vi "Shooter_SM.vi"   [LabVIEW 2017]
uses:
  Enum_Shooter_SM_State.ctl
  Enum_Shooter_SM_Action.ctl
  Globals/Global_STOP.vi
  Global_HoodSensorPosition.vi
  Global_CMDShooter.vi
  Global_ShooterCTRL.vi
  Enum_ShooterCMDS.ctl
  Cluster_ShooterCMDInput.ctl
  Vision/Enum_ Field Targets.ctl
  Vision/ENUM_Location Zones.ctl
  Vision/Cluster_HW Data Out.ctl
  Vision/Global_HW Data Out.vi
types:
  T1 = typedef "Vision.lvlib/Cluster_HW Data Out.ctl" = cluster{"Target Found":bool, "Target":T2, "Nominal to Center (-1to1":dbl, "Pixels to Center":dbl, "Vision Distance (in)":dbl, "Location":T3}
  T2 = typedef "Vision.lvlib/Enum_ Field Targets.ctl" = enum16{"None", "Peg", "Boiler", "Rope"}
  T3 = typedef "Vision.lvlib/ENUM_Location Zones.ctl" = enum16{"Unknown", "Close", "Medium-Close", "Medium", "Medium -Far", "Far"}
  T4 = typedef "Cluster_ShooterCMDInput.ctl" = cluster{"Fly Wheel Input":dbl, "Hood position Input":dbl, "CMD Mode":T5}
  T5 = typedef "Enum_ShooterCMDS.ctl" = enum16{"Shooting", "Not Shooting"}
  T6 = typedef "Enum_Shooter_SM_Action.ctl" = enum16{"No Action", "Reset Time", "Reset All", "Set Hood", "Set Fly Wheel", "Stop Hood"}
  T7 = typedef "Enum_Shooter_SM_State.ctl" = enum16{"Startup", "Idle", "Shutdown", "Check Position"}
  T8 = cluster{"Action":T6[], "State":T7, "Current Time":timestamp, "Start Time":timestamp, "Loop Time (ms)":u32, "Hood Position Out":dbl, "Fly Wheel Out":dbl, "Hood Sensor Position":dbl, "Shooter CMD":T4, "Hood VBus Out":dbl, "Hood Pos/Vbus":bool, "Tracking Data OUT":T1}
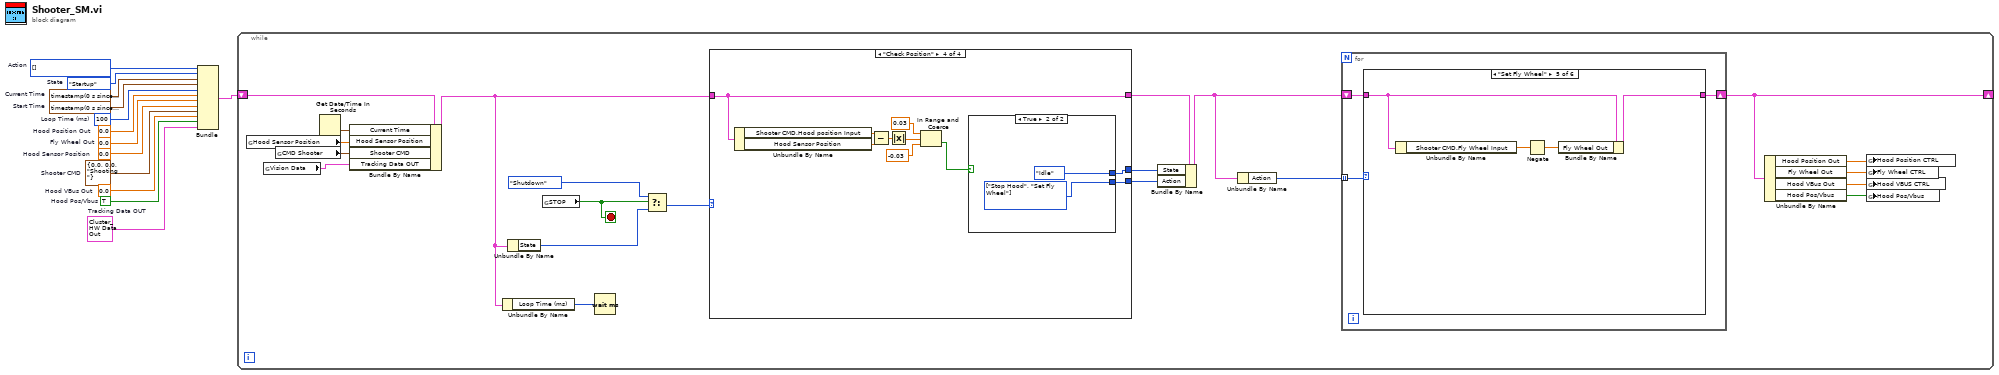
[diagram p0: block diagram]
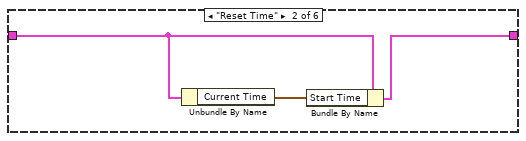
[diagram p3: hidden frame]
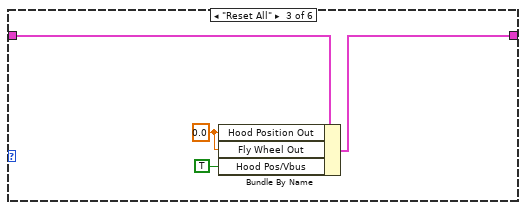
[diagram p4: hidden frame]
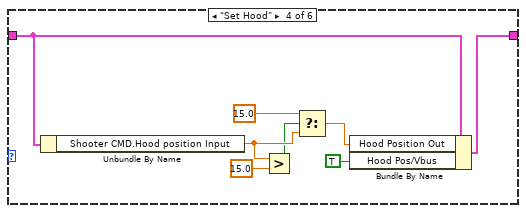
[diagram p5: hidden frame]
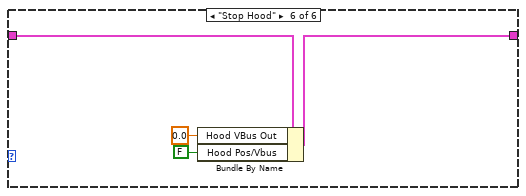
[diagram p6: hidden frame]
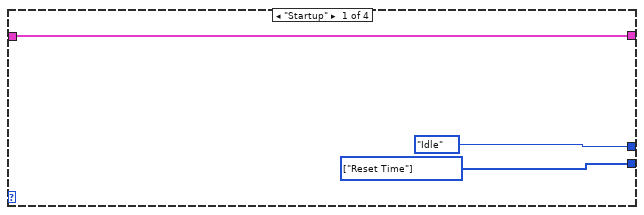
[diagram p7: hidden frame]
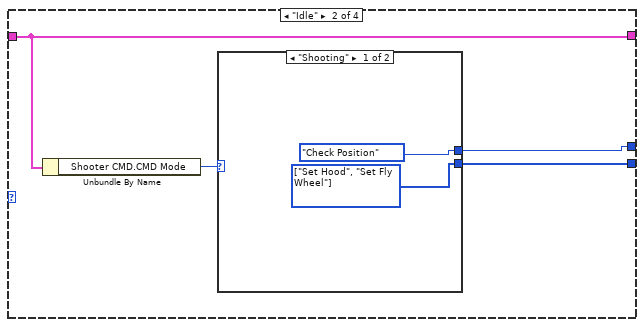
[diagram p8: hidden frame]
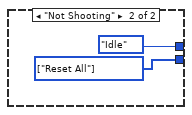
[diagram p9: hidden frame]
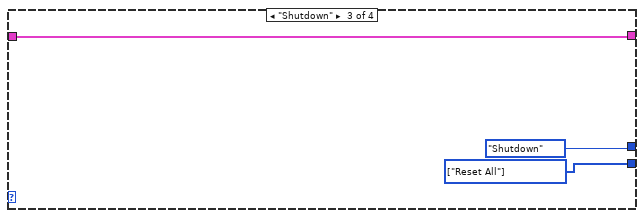
[diagram p10: hidden frame]
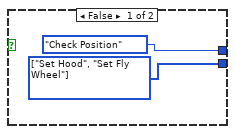
[diagram p11: hidden frame]
diagram:
  w1 = T1 {"Target Found"=FALSE, "Target"=enum."None", "Nominal to Center (-1to1"=0.0, "Pixels to Center"=0.0, "Vision Distance (in)"=0.0, "Location"=enum."Unknown"}  # Tracking Data OUT
  w13 = TRUE  # Hood Pos/Vbus
  w12 = 0.0  # Hood VBus Out
  w11 = T4 {"Fly Wheel Input"=0.0, "Hood position Input"=0.0, "CMD Mode"=enum."Shooting"}  # Shooter CMD
  w10 = 0.0  # Hood Sensor Position
  w9 = 0.0  # Fly Wheel Out
  w8 = 0.0  # Hood Position Out
  w7 = T6[] [] items=["No Action", "Reset Time", "Reset All", "Set Hood", "Set Fly Wheel", "Stop Hood"]  # Action
  w6 = Enum_Shooter_SM_State."Startup"  # State
  w2 = u32 100  # Loop Time (ms)
  w3 = timestamp(0 s since 1904-01-01)  # Start Time
  w4 = timestamp(0 s since 1904-01-01)  # Current Time
  n1 = Bundle("Action"=w7, "State"=w6, "Current Time"=w4, "Start Time"=w3, "Loop Time (ms)"=w2, "Hood Position Out"=w8, "Fly Wheel Out"=w9, "Hood Sensor Position"=w10, "Shooter CMD"=w11, "Hood VBus Out"=w12, "Hood Pos/Vbus"=w13, "Tracking Data OUT"=w1) -> (w5:T8)  [unwired: 1 in]
  n2 = while {
    shift-right: [w21] -> _
    shift-left: w5 -> [w26]
    stop <- w33 stop-if-true
    n3 = global read "Global_HoodSensorPosition.vi" "Hood Sensor Position"() -> (w24:dbl)
    n4 = global read "Global_HW Data Out.vi" "Vision Data"() -> (w14:T1)
    n5 = global read "Global_CMDShooter.vi" "CMD Shooter"() -> (w22:T4)
    n6 = Get Date/Time In Seconds() -> (seconds since 1Jan1904=w23:timestamp)
    n7 = Bundle By Name(cluster=w26, "Current Time"=w23, "Hood Sensor Position"=w24, "Shooter CMD"=w22, "Tracking Data OUT"=w14) -> (w25:T8)
    n8 = Unbundle By Name(w25) -> ("Loop Time (ms)"=w30:u32)
    n9 = Unbundle By Name(w25) -> ("State"=w31:T7)
    n10 = global read "Global_Stop.vi" "STOP"() -> (w33:bool)
    n11 = Wait (ms)(milliseconds to wait=w30) -> ()  [unwired: 1 out]
    n12 = Select(t=Enum_Shooter_SM_State."Shutdown" ("Enum"), s=w33, f=w31) -> (s? t:f=w34:T7)
    n13 = case shown="\"Check Position\"" w34 {
      tunnel: w25 -> [w62 w66 w73 w85]
      tunnel: [w62 w66 w73 w85] -> w29
      tunnel: [Enum_Shooter_SM_State."Idle" ("State") w68 Enum_Shooter_SM_State."Shutdown" ("State") w77] -> w18
      tunnel: [w63 w67 w74 w76] -> w17
      frame "Startup" {
        w63 = T6[] [enum."Reset Time"] items=["No Action", "Reset Time", "Reset All", "Set Hood", "Set Fly Wheel", "Stop Hood"] ("Action")
      }
      frame "Idle" {
        n14 = Unbundle By Name(w66) -> ("Shooter CMD.CMD Mode"=w65:T5)
        n15 = case shown="\"Shooting\"" w65 {
          tunnel: [Enum_Shooter_SM_State."Check Position" ("State") Enum_Shooter_SM_State."Idle" ("State")] -> w68
          tunnel: [w69 w71] -> w67
          frame "Shooting" {
            w69 = T6[] [enum."Set Hood", enum."Set Fly Wheel"] items=["No Action", "Reset Time", "Reset All", "Set Hood", "Set Fly Wheel", "Stop Hood"] ("Action")
          }
          frame "Not Shooting" {
            w71 = T6[] [enum."Reset All"] items=["No Action", "Reset Time", "Reset All", "Set Hood", "Set Fly Wheel", "Stop Hood"] ("Action")
          }
        }
      }
      frame "Shutdown" {
        w74 = T6[] [enum."Reset All"] items=["No Action", "Reset Time", "Reset All", "Set Hood", "Set Fly Wheel", "Stop Hood"] ("Action")
      }
      frame "Check Position" {
        n16 = Unbundle By Name(w85) -> ("Shooter CMD.Hood position Input"=w83:dbl, "Hood Sensor Position"=w84:dbl)
        n17 = Subtract(x=w83, y=w84) -> (x-y=w82:dbl)
        n18 = Absolute Value(x=w82) -> (abs(x)=w81:dbl)
        n19 = In Range and Coerce(upper limit=0.03, x=w81, lower limit=-0.03) -> (In Range?=w78:bool)  [unwired: 1 out]
        n20 = case shown="True" w78 {
          tunnel: [Enum_Shooter_SM_State."Check Position" ("State") Enum_Shooter_SM_State."Idle" ("State")] -> w77
          tunnel: [w86 w88] -> w76
          frame False {
            w86 = T6[] [enum."Set Hood", enum."Set Fly Wheel"] items=["No Action", "Reset Time", "Reset All", "Set Hood", "Set Fly Wheel", "Stop Hood"] ("Action")
          }
          frame True {
            w88 = T6[] [enum."Stop Hood", enum."Set Fly Wheel"] items=["No Action", "Reset Time", "Reset All", "Set Hood", "Set Fly Wheel", "Stop Hood"] ("Action")
          }
        }
      }
    }
    n21 = Bundle By Name(cluster=w29, "State"=w18, "Action"=w17) -> (w28:T8)
    n22 = Unbundle By Name(w28) -> ("Action"=w27:T6[])
    n23 = for {
      shift-right: [w35] -> w21
      shift-left: w28 -> [w36]
      tunnel: w27 -> [w37] mode=indexing
      n24 = case shown="\"Set Fly Wheel\"" w37 {
        tunnel: w36 -> [w38 w40 w45 w52 w57 w61]
        tunnel: [w38 w39 w44 w53 w56 w60] -> w35
        frame "No Action" {
        }
        frame "Reset Time" {
          n25 = Unbundle By Name(w40) -> ("Current Time"=w41:timestamp)
          n26 = Bundle By Name(cluster=w40, "Start Time"=w41) -> (w39:T8)
        }
        frame "Reset All" {
          w43 = 0.0 ("Hood Position Out")
          n27 = Bundle By Name(cluster=w45, "Hood Position Out"=w43, "Fly Wheel Out"=w43, "Hood Pos/Vbus"=TRUE) -> (w44:T8)
        }
        frame "Set Hood" {
          n28 = Unbundle By Name(w52) -> ("Shooter CMD.Hood position Input"=w49:dbl)
          n29 = Greater?(x=w49, y=15.0) -> (0:w47:bool)
          n30 = Select(t=15.0, s=w47, f=w49) -> (s? t:f=w48:dbl)
          n31 = Bundle By Name(cluster=w52, "Hood Position Out"=w48, "Hood Pos/Vbus"=TRUE) -> (w53:T8)
        }
        frame "Set Fly Wheel" {
          n32 = Unbundle By Name(w57) -> ("Shooter CMD.Fly Wheel Input"=w55:dbl)
          n33 = Negate(x=w55) -> (-x=w54:dbl)
          n34 = Bundle By Name(cluster=w57, "Fly Wheel Out"=w54) -> (w56:T8)
        }
        frame "Stop Hood" {
          n35 = Bundle By Name(cluster=w61, "Hood VBus Out"=0.0, "Hood Pos/Vbus"=FALSE) -> (w60:T8)
        }
      }
    }
    n36 = Unbundle By Name(w21) -> ("Hood Position Out"=w19:dbl, "Fly Wheel Out"=w20:dbl, "Hood VBus Out"=w16:dbl, "Hood Pos/Vbus"=w15:bool)
    n37 = global write "Global_ShooterCTRL.vi" "Hood Position CTRL"(w19) -> ()
    n38 = global write "Global_ShooterCTRL.vi" "Fly Wheel CTRL"(w20) -> ()
    n39 = global write "Global_ShooterCTRL.vi" "Hood VBUS CTRL"(w16) -> ()
    n40 = global write "Global_ShooterCTRL.vi" "Hood Pos/Vbus"(w15) -> ()
  }
